vi "Config Scaling.vi"(0 "VISA resource name":refnum<visa-resource-name>, 1 "Power Coefficient (1.000)":dbl=1.0 min=0.001 max=9999.0 step=0.001 format="%^.3e", 2 "CT Ratio (1.000)":dbl=1.0 min=0.001 max=9999.0 step=0.001 format="%^.3e", 3 "PT Ratio (1.000)":dbl=1.0 min=0.001 max=9999.0 step=0.001 format="%^.3e", 5 "Scaling (F: OFF)":bool, 7 "Element (0: All)":u16(ring) items=["ALL", "Element1", "Element2", "Element3"], 11 "error in (no error)":errorcluster) -> (4 "VISA resource name out":refnum<visa-resource-name>, 15 "error out":errorcluster)   [LabVIEW 2010, in "Yokogawa WT200 Series.lvlib"]
doc: "This VI sends the scaling commands to the WT200 Series."
uses:
  G:/Engineering/Retail/LabV/instr.lib/Yokogawa WT200 Series/Yokogawa WT200 Series.lvlib
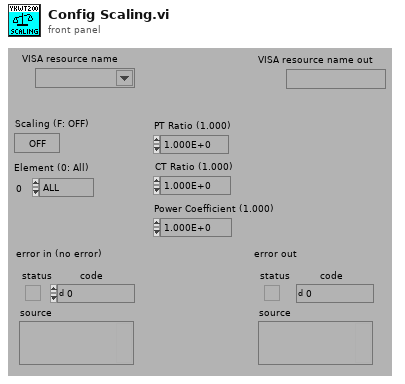
[diagram p1: front panel]
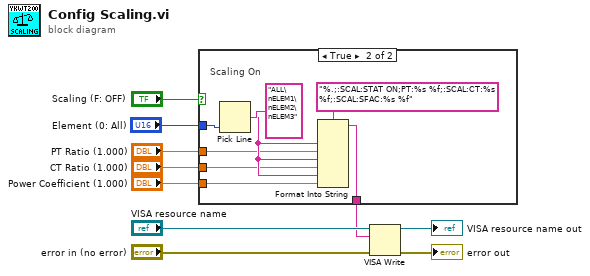
[diagram p0: block diagram]
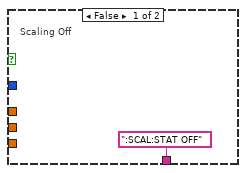
[diagram p2: hidden frame]
diagram:
  n1 = case shown="True" "Scaling (F: OFF)" {
    tunnel: [":SCAL:STAT OFF" w18] -> w2
    tunnel: "PT Ratio (1.000)" -> [_ w14]
    tunnel: "CT Ratio (1.000)" -> [_ w13]
    tunnel: "Power Coefficient (1.000)" -> [_ w12]
    tunnel: "Element (0: All)" -> [_ w16]
    frame False {
      # "Scaling Off"
    }
    frame True {
      # "Scaling On"
      n2 = Pick Line(multi-line string="ALL\nELEM1\nELEM2\nELEM3", line index=w16) -> (output string=w15:string)  [unwired: 1 in]
      n3 = Format Into String(format string="%.;:SCAL:STAT ON;PT:%s %f;:SCAL:CT:%s %f;:SCAL:SFAC:%s %f", w15, w14, w15, w13, w15, w12) -> (resulting string=w18:string)  [unwired: 2 in, 1 out]
    }
  }
  n4 = VISA Write(VISA resource name="VISA resource name", write buffer=w2, error in (no error)="error in (no error)") -> (VISA resource name out=→"VISA resource name out":refnum<visa-resource-name>, error out=→"error out":errorcluster)  [unwired: 1 out]
